vi "init.vi"(8 "error in":errorcluster, 10 "TBM module configuration in":refnum<class "TBM module configuration.lvclass">, 11 "Scan Engine runtime in":refnum<class "Scan Engine runtime.lvclass">) -> (0 "error out":errorcluster, 1 "data allocations":T1, 2 "execution settings":T4, 3 "Scan Engine runtime out":refnum<class "Scan Engine runtime.lvclass">)   [LabVIEW 2013, in "Scan Engine runtime.lvclass"]
doc: "Provides an interface for initializing a module at runtime. While this interface performs no operations, a child should provide an override which may open any necessary references or sessions, allocate necessary memory, and perform any final configuration validataion before providing the full configuration <b>execution data</b> to the calling process."
uses:
  Scan Engine runtime.lvclass
  <vilib>/NI/Tag Bus Module Framework/module configuration/TBM module configuration.lvclass
  <vilib>/NI/Tag Bus Module Framework/runtime/execution settings.ctl
  <vilib>/NI/Tag Bus Module Framework/channel/data tables.ctl
  <vilib>/NI/Tag Bus/dictionary/data dictionary.lvclass
  <vilib>/NI/Tag Bus/dictionary table pair.ctl
  <vilib>/NI/Tag Bus/table/data table.ctl
  configuration/Scan Engine configuration.lvclass
  Scan Engine runtime.lvclass/Scan Engine runtime.ctl
  Custom Ctrls/Index Map.ctl
  <vilib>/NI/Tag Bus/tag/Data Type.ctl
  <vilib>/NI/Tag Bus/tag/tag descriptor.lvclass/tag descriptor.ctl
  <vilib>/NI/Tag Bus Module Framework/channel/TBM channel.lvclass/TBM channel.ctl
  <vilib>/NI/Tag Bus Module Framework/channel/TBM channel.lvclass
  <vilib>/NI/Tag Bus Module Framework/runtime/TBM module execution interface.lvclass
  <vilib>/NI/Tag Bus/tag/tag descriptor.lvclass
  <vilib>/NI/Tag Bus/tag bus.lvlib
  <vilib>/NI/Tag Bus/table/data table.lvlib
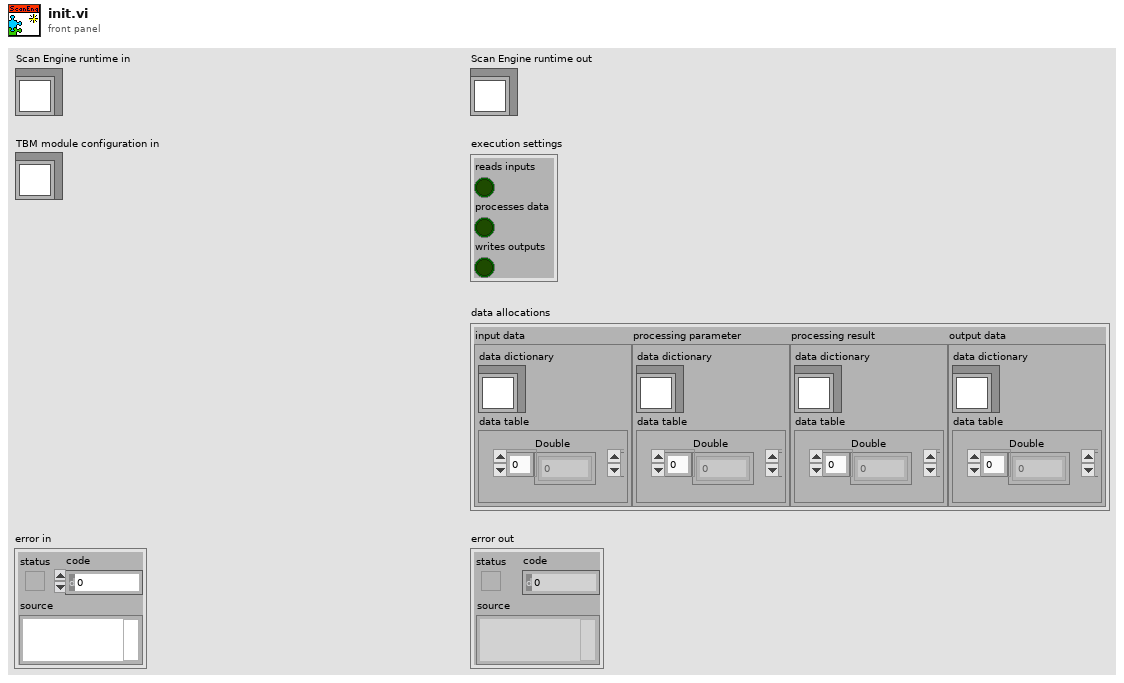
[diagram p1: front panel]
types:
  T1 = typedef "TBM channel.lvclass/data tables.ctl" = cluster{"input data":T2, "processing parameter":T2, "processing result":T2, "output data":T2}
  T2 = typedef "tag bus.lvlib/dictionary table pair.ctl" = cluster{"data dictionary":refnum<class "data dictionary.lvclass">, "data table":T3}
  T3 = typedef "tag bus.lvlib/data table.lvlib/data table.ctl" = cluster{"Double":dbl[], "Single":sgl[], "I64":i64[], "I32":i32[], "I16":i16[], "I8":i8[], "U64":u64[], "U32":u32[], "U16":u16[], "U8":u8[], "Boolean":bool[], "String":string[], "Array of Double":cluster{"DBL Array":dbl[]}[], "Array of Single":cluster{"SGL Array":sgl[]}[], "Array of I64":cluster{"I64 Array":i64[]}[], "Array of I32":cluster{"I32 Array":i32[]}[], "Array of I16":cluster{"I16 Array":i16[]}[], "Array of I8":cluster{"I8 Array":i8[]}[], "Array of U64":cluster{"U64 Array":u64[]}[], "Array of U32":cluster{"U32 Array":u32[]}[], "Array of U16":cluster{"U16 Array":u16[]}[], "Array of U8":cluster{"U8 Array":u8[]}[], "Array of Boolean":cluster{"Boolean Array":bool[]}[], "Array of String":cluster{"String Array":string[]}[]}
  T4 = typedef "TBM module execution interface.lvclass/execution settings.ctl" = cluster{"reads inputs":bool, "processes data":bool, "writes outputs":bool}
  T5 = typedef "Scan Engine runtime.lvclass/Index Map.ctl" = cluster{"data type":T6, "variable ref":refnum<k21>, "index":i32}
  T6 = typedef "tag bus.lvlib/tag descriptor.lvclass/Data Type.ctl" = enum16{"Double", "Single", "I64", "I32", "I16", "I8", "U64", "U32", "U16", "U8", "Boolean", "String", "Array of Double", "Array of Single", "Array of I64", "Array of I32", "Array of I16", "Array of I8", "Array of U64", "Array of U32", "Array of U16", "Array of U8", "Array of Boolean", "Array of String"}
  T7 = typedef "TBM channel.lvclass/channel classification.ctl" = enum16{"input data", "output data", "processing parameter", "processing result"}
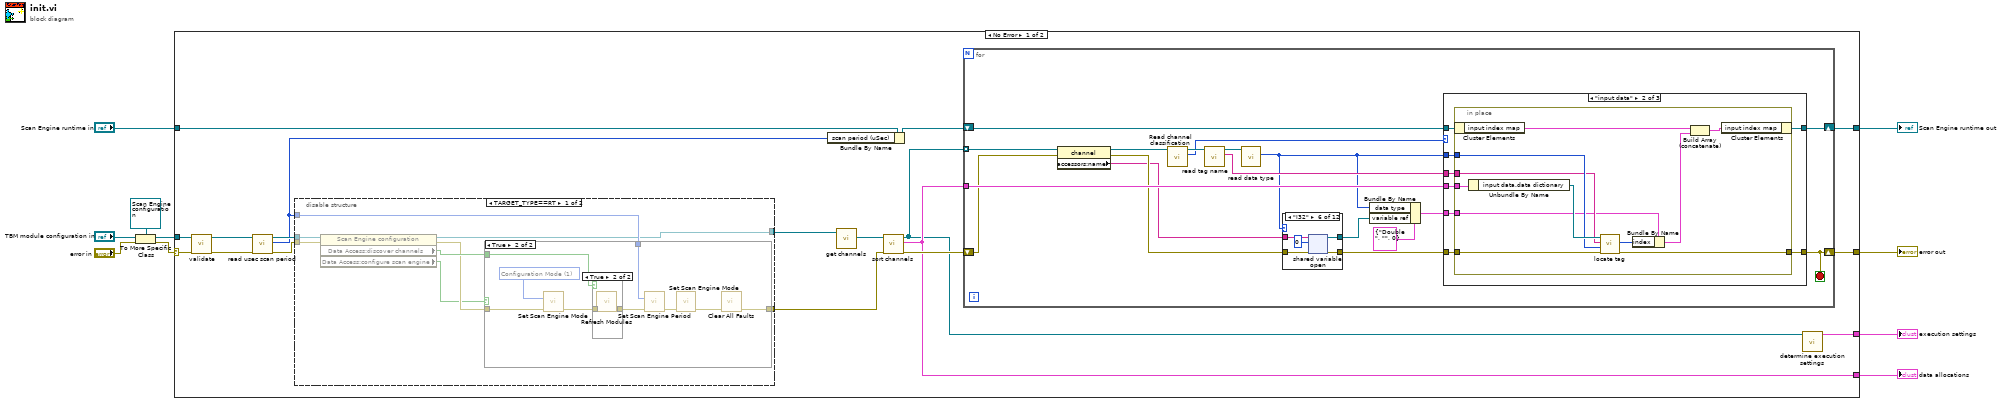
[diagram p0: block diagram]
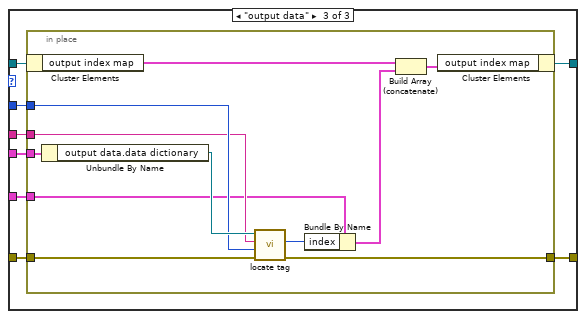
[diagram p6: hidden frame]
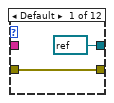
[diagram p7: hidden frame]
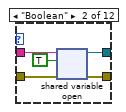
[diagram p8: hidden frame]
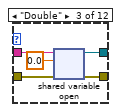
[diagram p9: hidden frame]
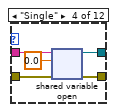
[diagram p10: hidden frame]
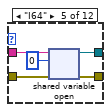
[diagram p11: hidden frame]
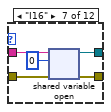
[diagram p12: hidden frame]
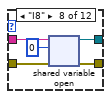
[diagram p13: hidden frame]
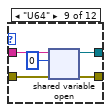
[diagram p14: hidden frame]
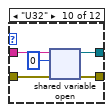
[diagram p15: hidden frame]
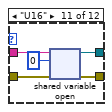
[diagram p16: hidden frame]
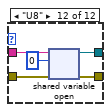
[diagram p17: hidden frame]
diagram:
  n1 = To More Specific Class(target class=refnum<class "Scan Engine configuration.lvclass"> refnum ("Synchronous module configuration"), reference="TBM module configuration in", error in="error in") -> (specific class reference=w9:refnum<class "Scan Engine configuration.lvclass">, error out=w10:errorcluster)
  n2 = case shown="No Error" w10 {
    selector: w10 -> [w27 w167]
    tunnel: w9 -> [w26 _]
    tunnel: "Scan Engine runtime in" -> [w25 w168]
    tunnel: [w24 w168] -> w4
    tunnel: [w22 w167] -> w1
    tunnel: [w21 _] -> w2
    tunnel: [w28 _] -> w3
    frame No Error {
      n3 = call-dynamic "validate.vi"("error in"=w27, "Scan Engine configuration in"=w26) -> ("error out"=w12:errorcluster, "Scan Engine configuration out"=w11:refnum<class "Scan Engine configuration.lvclass">)  [unwired: 8 in]
      n4 = call-dynamic "read usec scan period.vi"("error in"=w12, "Scan Engine configuration in"=w11) -> ("error out"=w16:errorcluster, "scan period (uSec)"=w15:u32, "Scan Engine configuration out"=w17:refnum<class "Scan Engine configuration.lvclass">)  [unwired: 7 in]
      n5 = disable-structure shown="TARGET_TYPE==RT" {
        disable-tunnel: [w36 w50] -> w18
        disable-tunnel: w17 -> [w35 w51]
        disable-tunnel: w16 -> [w34 w50]
        disable-tunnel: w15 -> [w33 _]
        disable-tunnel: [w30 w51] -> w14
        frame condition #0 {
          n6 = property class="Scan Engine configuration"(reference=w35, error in=w34) -> (reference out=w30:refnum<class "Scan Engine configuration.lvclass">, error out=w31:errorcluster, "Data Access:discover channels"=w32:bool, "Data Access:configure scan engine"=w29:bool)
          n7 = case shown="True" w29 {
            tunnel: [w37 w39] -> w36
            tunnel: w33 -> [_ w43]
            tunnel: w32 -> [_ w40]
            tunnel: w31 -> [w37 w42]
            frame False {
            }
            frame True {
              w41 = 1 items=["Configuration Mode"=1, "Active Mode"=2] ("mode (Active Mode)")
              n8 = call <vilib>:"Set Scan Engine Mode.vi"("mode (Active Mode)"=w41, "error in (no error)"=w42) -> ("error out"=w38:errorcluster)  [unwired: 13 in]
              n9 = case shown="True" w40 {
                tunnel: [w47 w49] -> w44
                tunnel: w38 -> [w47 w48]
                frame False {
                }
                frame True {
                  n10 = call <vilib>:"Refresh Modules.vi"("error in (no error)"=w48) -> ("error out"=w49:errorcluster)  [unwired: 10 in]
                }
              }
              n11 = call <vilib>:"Set Scan Engine Period.vi"("scan period (uSec)"=w43, "error in (no error)"=w44) -> ("error out"=w45:errorcluster)  [unwired: 13 in]
              n12 = call <vilib>:"Set Scan Engine Mode.vi"("error in (no error)"=w45) -> ("error out"=w46:errorcluster)  [unwired: 14 in]
              n13 = call <vilib>:"Clear All Faults.vi"("error in (no error)"=w46) -> ("error out"=w39:errorcluster)  [unwired: 10 in]
            }
          }
        }
        frame condition #1 (active) {
        }
      }
      n14 = Bundle By Name(cluster=w25, "scan period (uSec)"=w15) -> (w19:refnum<class "Scan Engine runtime.lvclass">)
      n15 = call-dynamic "get channels.vi"("module configuration in"=w14) -> ("channels"=w20:refnum<class "TBM channel.lvclass">[])  [unwired: 9 in, 1 out]
      n16 = call <vilib>:"sort channels.vi"("error in"=w18, "channels in"=w20) -> ("error out"=w23:errorcluster, "data allocations"=w21:T1, "channels out"=w13:refnum<class "TBM channel.lvclass">[])  [unwired: 7 in]
      n17 = for {
        shift-right: [w66] -> w24
        shift-left: w19 -> [w67]
        shift-right: [w59] -> w22
        shift-left: w23 -> [w62]
        tunnel: w13 -> [w58] mode=indexing
        tunnel: w21 -> [w69]
        stop <- w59 stop-if-true
        n18 = property class="channel"(reference=w58, error in=w62) -> (reference out=w61:refnum<class "TBM channel.lvclass">, error out=w60:errorcluster, "accessors:name"=w57:string)
        n19 = call <vilib>:"Read channel classification.vi"("channel in"=w61) -> ("channel classification"=w63:T7, "channel out"=w68:refnum<class "TBM channel.lvclass">)  [unwired: 8 in, 1 out]
        n20 = call <vilib>:"read tag name.vi"("system tag in"=w68) -> ("name"=w64:string, "system tag out"=w65:refnum<class "TBM channel.lvclass">)  [unwired: 8 in, 1 out]
        n21 = call <vilib>:"read data type.vi"("system tag in"=w65) -> ("data type"=w53:T6)  [unwired: 8 in, 2 out]
        n22 = case shown="\"I32\"" w53 {
          tunnel: w60 -> [w110 w116 w121 w126 w131 w136 w141 w146 w151 w156 w161 w166]
          tunnel: [w110 w115 w120 w125 w130 w135 w140 w145 w150 w155 w160 w165] -> w55
          tunnel: [refnum<k21> refnum w112 w118 w123 w129 w134 w139 w144 w149 w154 w159 w164] -> w56
          tunnel: w57 -> [_ w113 w119 w124 w127 w132 w137 w142 w147 w152 w157 w162]
          frame Default {
          }
          frame "Boolean" {
            n23 = shared-variable-open(w113, w116, TRUE) -> (w112:refnum<k21>, w115:errorcluster)  [unwired: 1 in]
          }
          frame "Double" {
            n24 = shared-variable-open(w119, w121, 0.0) -> (w118:refnum<k21>, w120:errorcluster)  [unwired: 1 in]
          }
          frame "Single" {
            n25 = shared-variable-open(w124, w126, sgl 0.0) -> (w123:refnum<k21>, w125:errorcluster)  [unwired: 1 in]
          }
          frame "I64" {
            n26 = shared-variable-open(w127, w131, i64 0) -> (w129:refnum<k21>, w130:errorcluster)  [unwired: 1 in]
          }
          frame "I32" {
            n27 = shared-variable-open(w132, w136, 0) -> (w134:refnum<k21>, w135:errorcluster)  [unwired: 1 in]
          }
          frame "I16" {
            n28 = shared-variable-open(w137, w141, i16 0) -> (w139:refnum<k21>, w140:errorcluster)  [unwired: 1 in]
          }
          frame "I8" {
            n29 = shared-variable-open(w142, w146, i8 0) -> (w144:refnum<k21>, w145:errorcluster)  [unwired: 1 in]
          }
          frame "U64" {
            n30 = shared-variable-open(w147, w151, u64 0) -> (w149:refnum<k21>, w150:errorcluster)  [unwired: 1 in]
          }
          frame "U32" {
            n31 = shared-variable-open(w152, w156, u32 0) -> (w154:refnum<k21>, w155:errorcluster)  [unwired: 1 in]
          }
          frame "U16" {
            n32 = shared-variable-open(w157, w161, u16 0) -> (w159:refnum<k21>, w160:errorcluster)  [unwired: 1 in]
          }
          frame "U8" {
            n33 = shared-variable-open(w162, w166, u8 0) -> (w164:refnum<k21>, w165:errorcluster)  [unwired: 1 in]
          }
        }
        n34 = Bundle By Name(cluster=T5 {"data type"=enum."Double", "variable ref"="", "index"=0} ("Runtime Mapping information"), "data type"=w53, "variable ref"=w56) -> (w54:T5)
        n35 = case shown="\"input data\"" w63 {
          tunnel: w69 -> [_ w79 w98]
          tunnel: w67 -> [w71 w78 w97]
          tunnel: [w71 w77 w96] -> w66
          tunnel: [w70 w76 w95] -> w59
          tunnel: w64 -> [_ w75 w94]
          tunnel: w55 -> [w70 w74 w93]
          tunnel: w54 -> [_ w73 w92]
          tunnel: w53 -> [_ w72 w91]
          frame Default {
          }
          frame "input data" {
            n36 = in-place {
              in-place-border: w79 -> [w90]
              in-place-border: w75 -> [w84]
              in-place-border: w72 -> [w85]
              in-place-border: w74 -> [w83]
              in-place-border: w73 -> [w82]
              in-place-border: [w81] -> w76
              n37 = in-place-cluster #1(w78) -> ("input index map"=w88:T5[])
              n38 = Unbundle By Name(w90) -> ("input data.data dictionary"=w89:refnum<class "data dictionary.lvclass">)
              n39 = call <vilib>:"locate tag.vi"("error in"=w83, "data type"=w85, "name"=w84, "data dictionary in"=w89) -> ("error out"=w81:errorcluster, "index"=w86:i32)  [unwired: 5 in, 1 out]
              n40 = Bundle By Name(cluster=w82, "index"=w86) -> (w80:T5)
              n41 = Build Array (concatenate)(w88, w80) -> (w87:T5[])
              n42 = in-place-cluster #1("input index map"=w87) -> (w77:refnum<class "Scan Engine runtime.lvclass">)
            }
          }
          frame "output data" {
            n43 = in-place {
              in-place-border: w98 -> [w109]
              in-place-border: w94 -> [w103]
              in-place-border: w91 -> [w104]
              in-place-border: w93 -> [w102]
              in-place-border: w92 -> [w101]
              in-place-border: [w100] -> w95
              n44 = in-place-cluster #2(w97) -> ("output index map"=w107:T5[])
              n45 = Unbundle By Name(w109) -> ("output data.data dictionary"=w108:refnum<class "data dictionary.lvclass">)
              n46 = call <vilib>:"locate tag.vi"("error in"=w102, "data type"=w104, "name"=w103, "data dictionary in"=w108) -> ("error out"=w100:errorcluster, "index"=w105:i32)  [unwired: 5 in, 1 out]
              n47 = Bundle By Name(cluster=w101, "index"=w105) -> (w99:T5)
              n48 = Build Array (concatenate)(w107, w99) -> (w106:T5[])
              n49 = in-place-cluster #2("output index map"=w106) -> (w96:refnum<class "Scan Engine runtime.lvclass">)
            }
          }
        }
      }
      n50 = call <vilib>:"determine execution settings.vi"("channels"=w13) -> ("execution settings"=w28:T4)  [unwired: 10 in]
    }
    frame Error {
    }
  }
  "error out" <- w1
  "Scan Engine runtime out" <- w4
  "execution settings" <- w3
  "data allocations" <- w2
